vi "Configuration Process.vi"(8 "error in (no error)":errorcluster, 11 "View Model":T1) -> (0 "error out":errorcluster)   [LabVIEW 2017]
doc: "Handles all read/write to configuration file."
uses:
  View Model/Controls/View Model.ctl
  Error Handler/Controls/Error Model.ctl
  Error Handler/Controls/Error Type.ctl
  View Model/Controls/Shared Model.ctl
  Elevator Controller/Controls/Elevator Model.ctl
  Elevator Controller/Controls/Controller Overhead.ctl
  Elevator Controller/Controls/Elevator Commands.ctl
  Controls/Configuration Model.ctl
  Controls/Configuration Data.ctl
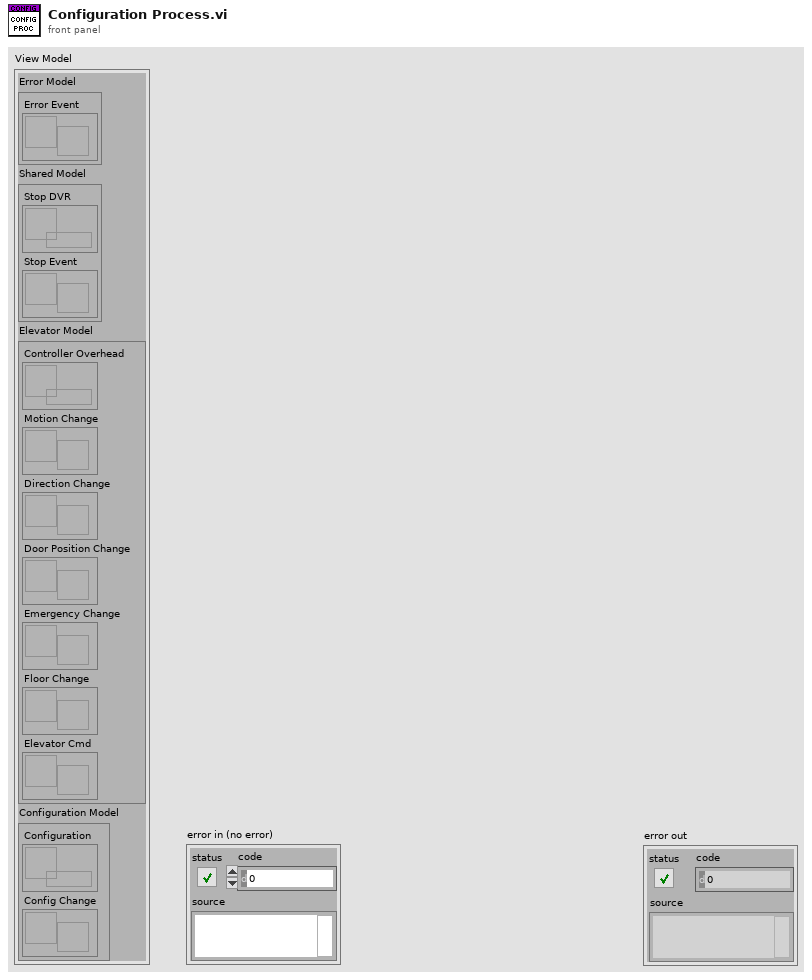
[diagram p1: front panel]
types:
  T1 = typedef "View Model.ctl" = cluster{"Error Model":T2, "Shared Model":T3, "Elevator Model":T4, "Configuration Model":T5}
  T2 = typedef "Error Model.ctl" = cluster{"Error Event":refnum<user-event>}
  T3 = typedef "Shared Model.ctl" = cluster{"Stop DVR":refnum<data-value>, "Stop Event":refnum<user-event>}
  T4 = typedef "Elevator Model.ctl" = cluster{"Controller Overhead":refnum<data-value>, "Motion Change":refnum<user-event>, "Direction Change":refnum<user-event>, "Door Position Change":refnum<user-event>, "Emergency Change":refnum<user-event>, "Floor Change":refnum<user-event>, "Elevator Cmd":refnum<user-event>}
  T5 = typedef "Configuration Model.ctl" = cluster{"Configuration":refnum<data-value>, "Config Change":refnum<user-event>}
  T6 = typedef "Configuration Data.ctl" = cluster{"Door Open":dbl, "Door Close":dbl, "Travel Time":dbl, "Inactivity Time":dbl}
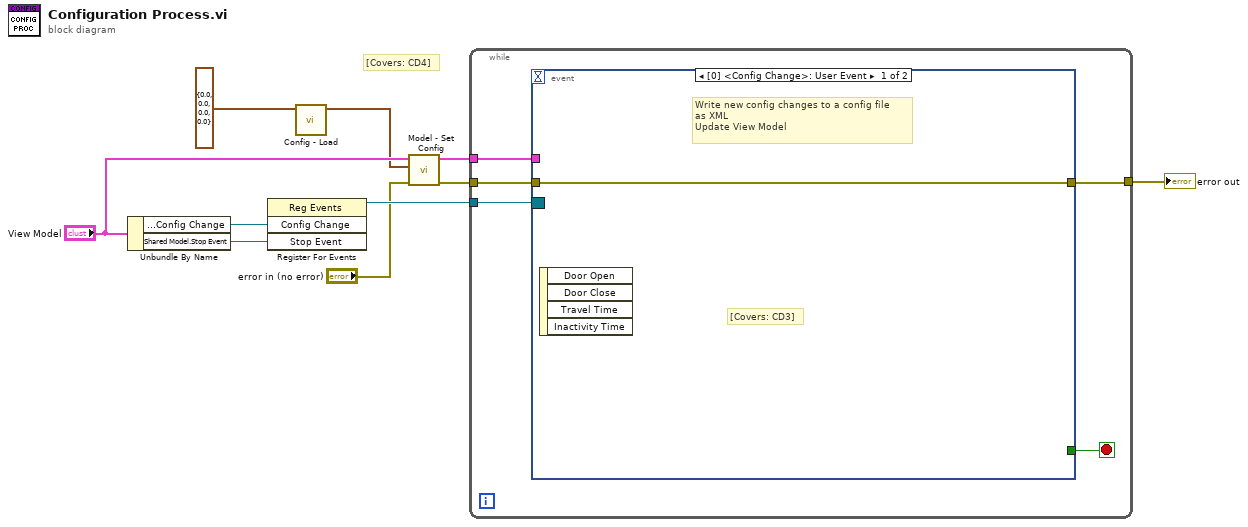
[diagram p0: block diagram]
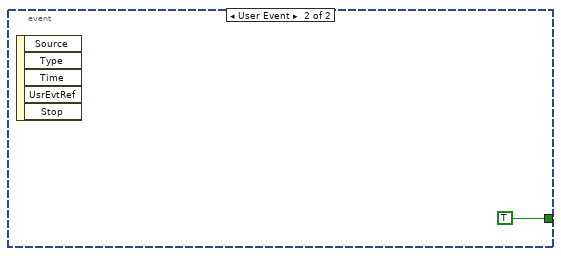
[diagram p2: hidden frame]
diagram:
  # "[Covers: CD4]"
  n1 = Unbundle By Name("View Model") -> ("Configuration Model.Config Change"=w9:refnum<user-event>, "Shared Model.Stop Event"=w8:refnum<user-event>)
  n2 = register-events(w9, w8) -> (reference out=w7:refnum<event-registration>)  [unwired: 2 in, 1 out]
  n3 = call "Config - Load.vi"("Default Configuration"=T6 {"Door Open"=0.0, "Door Close"=0.0, "Travel Time"=0.0, "Inactivity Time"=0.0}) -> ("Configuration"=w4:T6)  [unwired: 9 in, 1 out]
  n4 = call "Model - Set Config.vi"("error in (no error)"="error in (no error)", "Configuration"=w4, "View Model"="View Model") -> ("error out"=w2:errorcluster, "View Model"=w5:T1)  [unwired: 7 in]
  n5 = while {
    tunnel: w7 -> [w15]
    tunnel: w5 -> [w14]
    tunnel: w2 -> [w12]
    tunnel: [w11] -> w1
    stop <- w13 stop-if-true
    n6 = event shown="[0] <Config Change>: User Event" {
      selector: w15 -> [_ _]
      dyn-events: _ -> [_ _]
      timeout: _ -> [_ _]
      tunnel: w14 -> [_ _]
      tunnel: [_ TRUE] -> w13
      tunnel: w12 -> [w16 _]
      tunnel: [w16 _] -> w11
      event User Event {
        # "[Covers: CD3]"
        # "Write new config changes to a config file\nas XML\nUpdate View Model"
        n7 = event-data() -> ()  [unwired: 1 in, 4 out]
      }
      event User Event {
        n8 = event-data() -> ()  [unwired: 1 in, 5 out]
      }
    }
  }
  "error out" <- w1
